vi "Create Missing Install Folders.vi"(8 "Error In":errorcluster, 11 "Configuration":T1) -> (0 "Error Out":errorcluster, 3 "Configuration":T1)   [LabVIEW 2011, in "LVH-Build-Tools.lvlib"]
doc: "This VI creates folders in the install directory to match the folder hierarchy in the source directory."
uses:
  <vilib>/LabVIEW Hacker/Build Tools/LVH-Build-Tools.lvlib
  Type Defs/Configuration.ctl
  Type Defs/Install Configuration.ctl
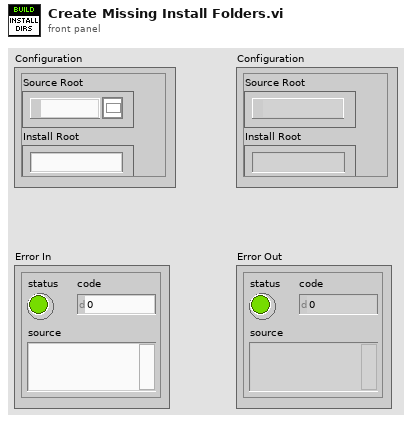
[diagram p1: front panel]
types:
  T1 = typedef "LVH-Build-Tools.lvlib/Configuration.ctl" = cluster{"Source Root":path, "Install Root":string, "Components":string[], "Ignore":string[], "Config Files":path[], "LV Directories":path[], "Install Paths":T2}
  T2 = typedef "LVH-Build-Tools.lvlib/Install Configuration.ctl" = cluster{"LabVIEW Directory":path, "Project Source Config":path}
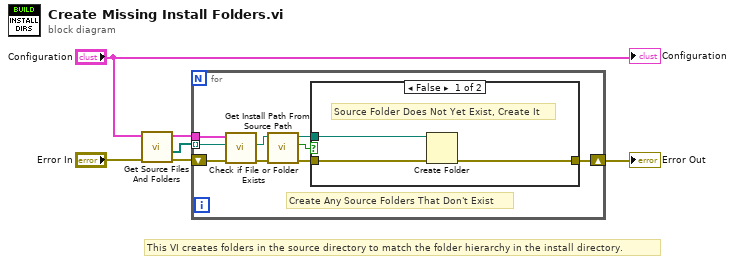
[diagram p0: block diagram]
diagram:
  # "This VI creates folders in the source directory to match the folder hierarchy in the install directory."
  n1 = call "Get Source Files And Folders.vi"("Error In"="Error In", "Configuration"="Configuration") -> ("Error Out"=w4:errorcluster, "All Source Folders"=w1:path[], "Configuration"=w2:T1)  [unwired: 6 in, 1 out]
  n2 = for {
    shift-right: [w12] -> w6
    shift-left: w4 -> [w10]
    tunnel: w2 -> [w8]
    tunnel: w1 -> [w7] mode=indexing
    # "Create Any Source Folders That Don't Exist"
    n3 = call "Get Install Path From Source Path.vi"("Error In"=w10, "Source File Path"=w7, "Configuration"=w8) -> ("Error Out"=w11:errorcluster, "Install File Path"=w9:path)  [unwired: 5 in, 2 out]
    n4 = call <vilib>:"Check if File or Folder Exists.vi"("error in (no error)"=w11, "path"=w9) -> ("error out"=w13:errorcluster, "file or folder exists?"=w15:bool, "dup path"=w14:path)  [unwired: 7 in]
    n5 = case shown="False" w15 {
      tunnel: w14 -> [w16 _]
      tunnel: w13 -> [w18 w19]
      tunnel: [w17 w19] -> w12
      frame False {
        # "Source Folder Does Not Yet Exist, Create It"
        n6 = Create Folder(path (use dialog)=w16, error in=w18) -> (error out=w17:errorcluster)  [unwired: 1 in, 2 out]
      }
      frame True {
        # "Source Folder Already Exists"
      }
    }
  }
  "Error Out" <- w6
  "Configuration" <- "Configuration"
